vi "GRAFOS.vi"() -> ()   [LabVIEW 2020]
uses:
  <vilib>/measure/NI_MABase.lvlib
panel:
  in  "FRECUENCIA":dbl(slide) scale=0.0..10.0
  in  "AMPLITUD":dbl(slide) scale=0.0..220.0
  in  "stop":bool
  out "Waveform Chart 4":waveform(dbl)(graph)
  out "Waveform Chart 3":waveform(dbl)(graph)
  out "Waveform Chart 2":waveform(dbl)(graph)
  out "Waveform Chart":waveform(dbl)(graph)
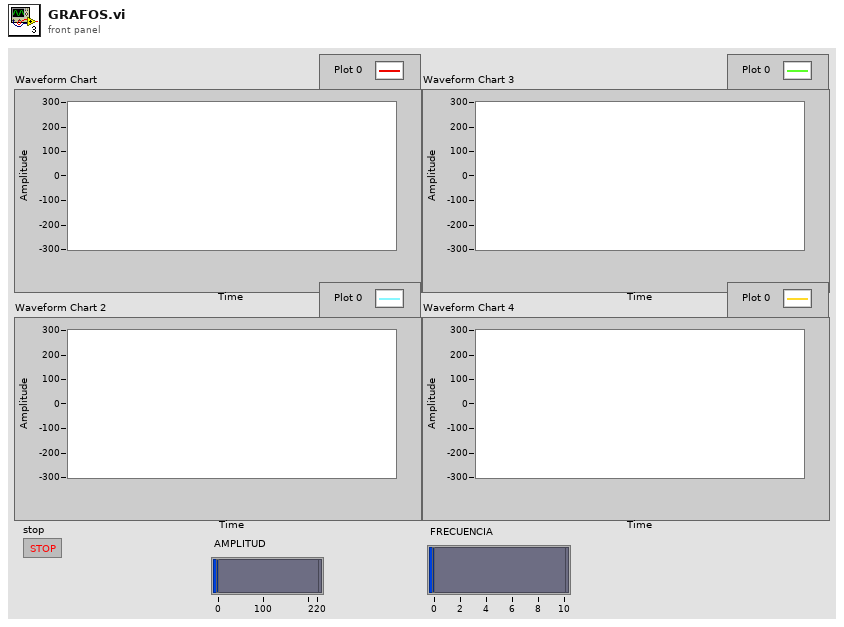
[diagram p1: front panel]
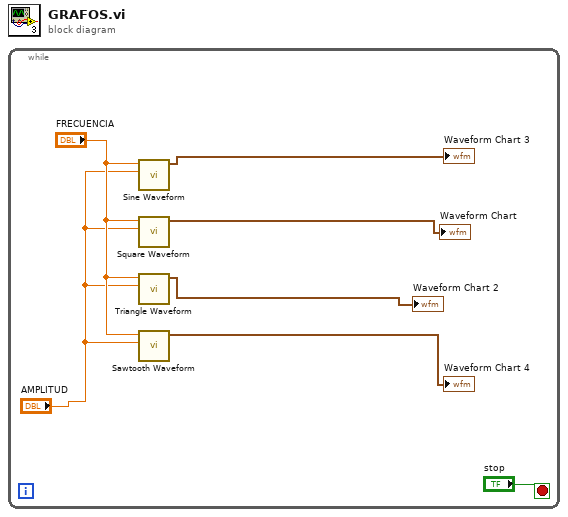
[diagram p0: block diagram]
diagram:
  n1 = while {
    stop <- "stop" stop-if-true
    n2 = call <vilib>:"Sine Waveform.vi"("amplitude"="AMPLITUD", "frequency"="FRECUENCIA") -> ("signal out"=→"Waveform Chart 3":waveform(dbl))  [unwired: 8 in, 1 out]
    n3 = call <vilib>:"Square Waveform.vi"("amplitude"="AMPLITUD", "frequency"="FRECUENCIA") -> ("signal out"=→"Waveform Chart":waveform(dbl))  [unwired: 8 in, 1 out]
    n4 = call <vilib>:"Triangle Waveform.vi"("amplitude"="AMPLITUD", "frequency"="FRECUENCIA") -> ("signal out"=→"Waveform Chart 2":waveform(dbl))  [unwired: 8 in, 1 out]
    n5 = call <vilib>:"Sawtooth Waveform.vi"("amplitude"="AMPLITUD", "frequency"="FRECUENCIA") -> ("signal out"=→"Waveform Chart 4":waveform(dbl))  [unwired: 8 in, 1 out]
  }
